vi "Get PhysChan.Commands.vi"(8 "error in (no error)":errorcluster, 11 "SLSC Interface in":refnum<class "SLSC Interface.lvclass">) -> (0 "error out":errorcluster, 2 "PhysChan.Commands":refnum<k21>[](array[refnum]), 3 "SLSC Interface out":refnum<class "SLSC Interface.lvclass">)   [LabVIEW 2015]
uses:
  SLSC Interface.lvclass
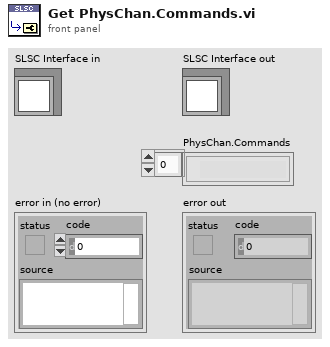
[diagram p1: front panel]
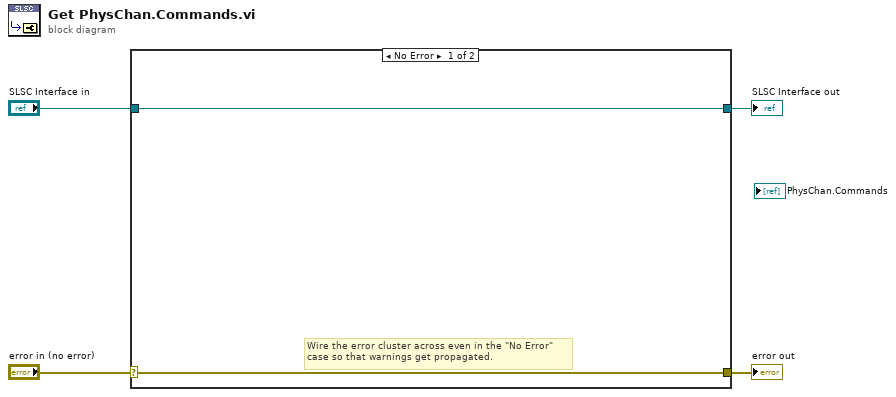
[diagram p0: block diagram]
diagram:
  n1 = case shown="No Error" "error in (no error)" {
    selector: "error in (no error)" -> [w6 w8]
    tunnel: [w6 w8] -> w3
    tunnel: [w5 w7] -> w1
    tunnel: "SLSC Interface in" -> [w5 w7]
    frame No Error {
      # "Wire the error cluster across even in the \"No Error\"\ncase so that warnings get propagated."
    }
    frame Error {
    }
  }
  "error out" <- w3
  "SLSC Interface out" <- w1
